vi "F16.vi"(8 "error in":errorcluster, 9 "data":u8[](array[numeric]), 10 "function":u8, 11 "device data model in":refnum<class "Standard Data Model.lvclass">) -> (0 "error out":errorcluster, 1 "data return":u8[](array[numeric]), 2 "function return":u8, 3 "device data model out":refnum<class "Standard Data Model.lvclass">)   [LabVIEW 2013, in "Modbus Library - Advance.lvlib" / "Standard Data Model.lvclass"]
doc: "Executes function code 16"
uses:
  Standard Data Model.lvclass
  Modbus Library - Advance.lvlib
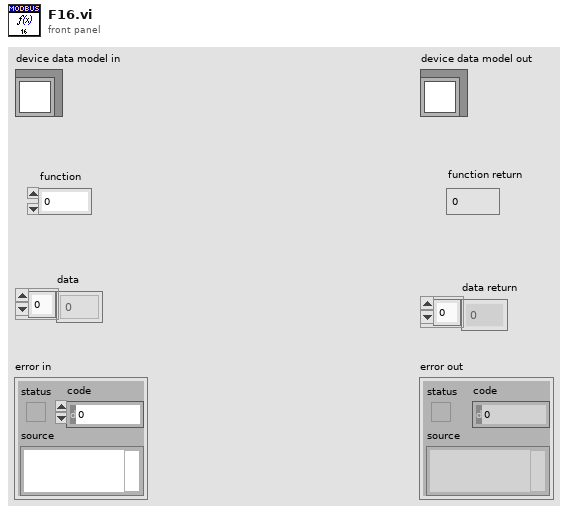
[diagram p1: front panel]
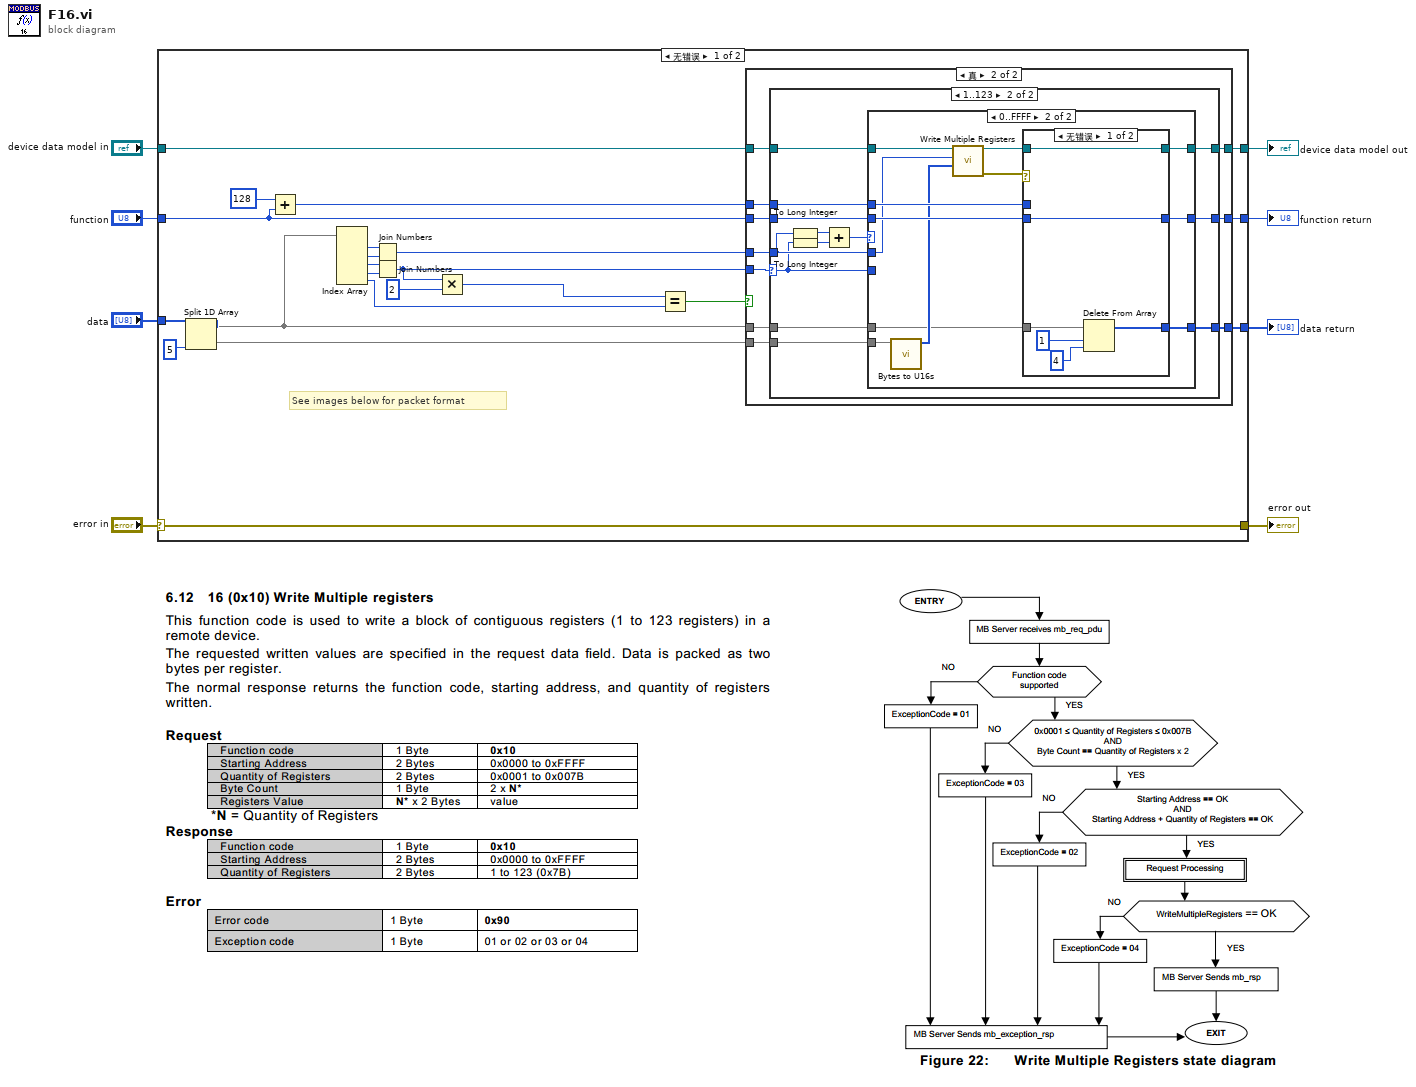
[diagram p0: block diagram]
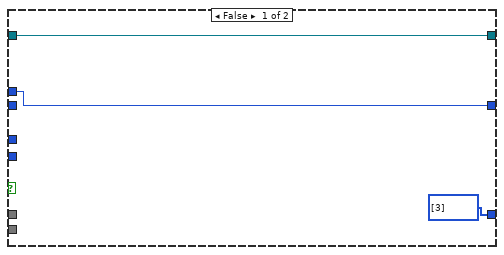
[diagram p2: hidden frame]
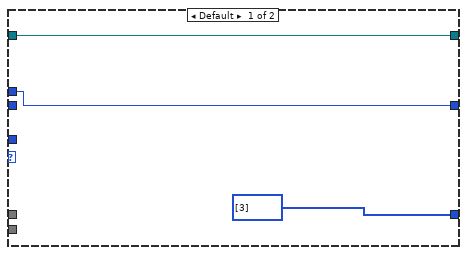
[diagram p3: hidden frame]
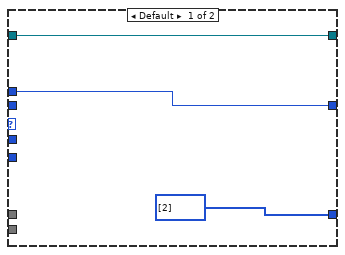
[diagram p4: hidden frame]
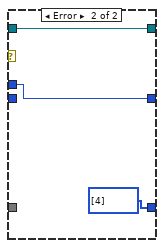
[diagram p5: hidden frame]
diagram:
  n1 = case shown="无错误" "error in" {
    selector: "error in" -> [w30 w87]
    tunnel: [w30 w87] -> w7
    tunnel: [w25 w86] -> w5
    tunnel: "device data model in" -> [w24 w86]
    tunnel: "function" -> [w21 w85]
    tunnel: "data" -> [w15 w84]
    tunnel: [w20 w85] -> w2
    tunnel: [w19 w84] -> w1
    frame No Error {
      # "See images below for packet format"
      n2 = Split 1D Array(array=w15, index=5) -> (first subarray=w12:u8[], second subarray=w13:u8[])
      n3 = Add(x=u8 128, y=w21) -> (x+y=w22:u8)
      n4 = Index Array(array=w12) -> (element #1=w28:u8, element #2=w29:u8, element #3=w27:u8, element #4=w26:u8, element #5=w10:u8)  [unwired: 5 in]
      n5 = Join Numbers(hi=w28, lo=w29) -> ((hi.lo)=w18:u16)
      n6 = Join Numbers(hi=w27, lo=w26) -> ((hi.lo)=w17:u16)
      n7 = Multiply(x=w17, y=u16 2) -> (x*y=w9:u16)
      n8 = Equal?(x=w9, y=w10) -> (x = y?=w11:bool)
      n9 = case shown="真" w11 {
        tunnel: w17 -> [_ w43]
        tunnel: [w33 w42] -> w25
        tunnel: w24 -> [w33 w41]
        tunnel: w22 -> [w32 w40]
        tunnel: w21 -> [_ w39]
        tunnel: [w32 w38] -> w20
        tunnel: [u8[] [3] ("Data Return") w37] -> w19
        tunnel: w18 -> [_ w36]
        tunnel: w13 -> [_ w35]
        tunnel: w12 -> [_ w34]
        frame False {
        }
        frame True {
          n10 = case shown="1..123" w43 {
            selector: w43 -> [_ w55]
            tunnel: [w46 w54] -> w42
            tunnel: w41 -> [w46 w53]
            tunnel: w40 -> [w45 w52]
            tunnel: w39 -> [_ w50]
            tunnel: [w45 w51] -> w38
            tunnel: [u8[] [3] ("Data Return") w49] -> w37
            tunnel: w36 -> [_ w56]
            tunnel: w35 -> [_ w48]
            tunnel: w34 -> [_ w47]
            frame Default {
            }
            frame 1..123 {
              n11 = To Long Integer(number=w56) -> (32bit integer=w59:i32)
              n12 = To Long Integer(number=w55) -> (32bit integer=w58:i32)
              n13 = Add(x=w59, y=w58) -> (x+y=w57:i32)
              n14 = case shown="0..FFFF" w57 {
                tunnel: w56 -> [_ w67]
                tunnel: w55 -> [_ _]
                tunnel: [w62 w74] -> w54
                tunnel: w53 -> [w62 w69]
                tunnel: w52 -> [w61 w73]
                tunnel: [w61 w71] -> w51
                tunnel: w50 -> [_ w72]
                tunnel: [u8[] [2] ("Data Return") w70] -> w49
                tunnel: w48 -> [_ w66]
                tunnel: w47 -> [_ w64]
                frame Default {
                }
                frame 0..65535 {
                  n15 = call "Bytes to U16s.vi"("Bytes"=w66) -> ("Registers"=w65:u16[])  [unwired: 10 in]
                  n16 = call-dynamic "Write Multiple Registers.vi"("register values"=w65, "starting address"=w67, "device data model in"=w69) -> ("error out"=w63:errorcluster, "device data model out"=w68:refnum<class "Standard Data Model.lvclass">)  [unwired: 7 in]
                  n17 = case shown="无错误" w63 {
                    tunnel: w68 -> [w80 w83]
                    tunnel: [w80 w83] -> w74
                    tunnel: w73 -> [_ w82]
                    tunnel: w72 -> [w79 _]
                    tunnel: [w79 w82] -> w71
                    tunnel: [w75 u8[] [4]] -> w70
                    tunnel: w64 -> [w78 _]
                    frame No Error {
                      n18 = Delete From Array(array=w78, length=1, index=4) -> (array with subset deleted=w75:u8[])  [unwired: 1 out]
                    }
                    frame Error {
                    }
                  }
                }
              }
            }
          }
        }
      }
    }
    frame Error {
    }
  }
  "error out" <- w7
  "device data model out" <- w5
  "data return" <- w1
  "function return" <- w2
